vi "Enumerate.vi"(8 "Error In":errorcluster, 11 "reference in":refnum<class "BubbleTeaShop.lvclass">) -> (0 "Error Out":errorcluster, 2 "ConsoleText":string, 3 "reference out":refnum<class "BubbleTeaShop.lvclass">)   [LabVIEW 2020, in "BubbleTeaShop.lvclass"]
uses:
  BubbleTeaShop.lvclass
  IBeverage_interface/IBeverage.lvclass
  Console_class/Console.lvclass
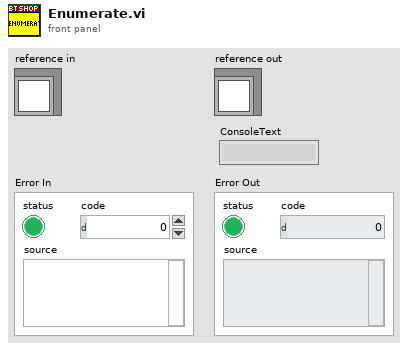
[diagram p1: front panel]
types:
  T1 = typedef "BubbleTeaShop.lvclass/ObjectAttributes.ctl" = cluster{"TakeAwayOrders":refnum<class "IBeverage.lvclass">[]}
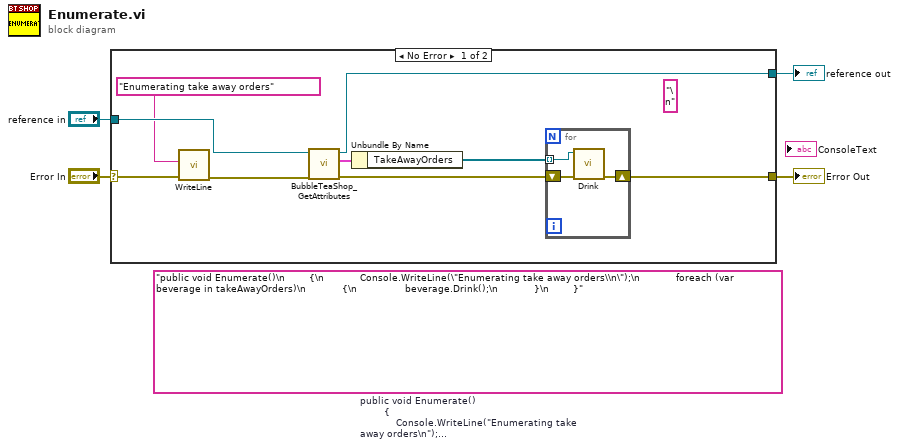
[diagram p0: block diagram]
diagram:
  (unwired) "public void Enumerate()\n        {\n            Console.WriteLine(\"Enumerating take away orders\\n\");\n            foreach (var beverage in takeAwayOrders)\n            {\n                beverage.Drink();\n            }\n        }"  # public void Enumerate()         {             Console.WriteLine("Enumerating take away orders\n");             foreach (var beverage in takeAwayOrders)             {                 beverage.Drink();             }         }
  n1 = case shown="No Error" "Error In" {
    selector: "Error In" -> [w7 w18]
    tunnel: [w8 w18] -> w3
    tunnel: [w12 w17] -> w1
    tunnel: "reference in" -> [w13 w17]
    frame No Error {
      (unwired) "\n" ("delimiter (Tab)")
      n2 = call "WriteLine.vi"("Error In"=w7, "ConsoleText"="Enumerating take away orders" ("delimiter (Tab)")) -> ("Error Out"=w6:errorcluster)  [unwired: 9 in]
      n3 = call "BubbleTeaShop_GetAttributes.vi"("error in (no error)"=w6, "reference in"=w13) -> ("error out"=w10:errorcluster, "Data"=w11:T1, "reference out"=w12:refnum<class "BubbleTeaShop.lvclass">)  [unwired: 6 in, 1 out]
      n4 = Unbundle By Name(w11) -> ("TakeAwayOrders"=w9:refnum<class "IBeverage.lvclass">[])
      n5 = for {
        tunnel: w9 -> [w15] mode=indexing
        shift-right: [w14] -> w8
        shift-left: w10 -> [w16]
        n6 = call-dynamic "Drink.vi"("Error In"=w16, "object in"=w15) -> ("Error Out"=w14:errorcluster)  [unwired: 8 in, 1 out]
      }
    }
    frame Error {
    }
  }
  "Error Out" <- w3
  "reference out" <- w1
